vi "DP.vi"(7 "Cluster 2":T1={{[44.26, 44.35, 44.44, 44.4, 44.32, 44.24, 44.13, 44.04, 43.96, 43.84, 43.81, 43.85, 43.72, 43.660000000000004, 43.730000000000004, 43.800000000000004, 43.93, 44.1, 44.22, 44.35, 44.47, 44.59, 44.800000000000004, 44.79, 44.82, 44.9, 45.02, 45.14, 45.35, 45.47, 45.59, 45.72, 45.88, 46.04, 46.0, 46.06, 46.13, 46.26, 46.42, 46.54, 46.67, 46.75, 46.83, 46.96, 47.08, 46.99, 47.03, 47.08, 47.160000000000004, 47.24, 47.32, 47.4, 47.49, 47.57, 47.65, 47.82, 47.730000000000004, 47.76, 47.84, 47.910000000000004, 47.99, 48.06, 48.14, 48.300000000000004, 48.43, 48.550000000000004, 48.67, 48.58, 48.6, 48.660000000000004, 48.75, 48.83, 48.94, 49.03, 49.11, 49.19, 49.27, 49.34, 49.2, 49.19, 49.230000000000004, 49.300000000000004, 49.35, 49.410000000000004, 49.57, 49.620000000000005, 49.660000000000004, 49.74, 49.57, 49.56, 49.58, 49.59, 49.620000000000005, 49.620000000000005, 49.660000000000004, 49.72, 49.75, 49.75, 49.76, 49.63, 49.63, 49.65, 49.65, 49.68, 49.71, 49.75, 49.78, 49.79, 49.870000000000005, 49.86, 49.7, 49.74, 49.75, 49.76, 49.81, 49.81, 49.86, 49.92, 49.97, 49.99, 50.0, 49.86, 49.86], [8.77817e-16, 8.28027e-16, 6.52256e-16, 7.37271e-16, 6.27782e-16, 7.80488e-16, 6.90707e-16, 8.78684e-16, 6.40232e-16, 7.51014e-16, 8.39314e-16, 7.48335e-16, 8.32474e-16, 7.10942e-16, 8.13954e-16, 7.61842e-16, 7.02305e-16, 8.45773e-16, 8.03435e-16, 9.26691e-16, 7.76441e-16, 8.47353e-16, 7.63208e-16, 7.75768e-16, 6.68938e-16, 6.3854e-16, 7.55169e-16, 9.2689e-16, 6.32594e-16, 7.8272e-16, 7.1802e-16, 7.55778e-16, 7.51571e-16, 7.70614e-16, 8.06029e-16, 8.48296e-16, 7.03956e-16, 8.42624e-16, 9.30632e-16, 6.06052e-16, 6.08322e-16, 7.13091e-16, 7.19724e-16, 7.89003e-16, 7.39076e-16, 8.69906e-16, 8.07947e-16, 7.16363e-16, 7.4837e-16, 8.39116e-16, 7.669e-16, 7.29213e-16, 7.26208e-16, 7.54206e-16, 9.32708e-16, 6.57226e-16, 8.41261e-16, 8.58932e-16, 7.73647e-16, 8.51593e-16, 9.21785e-16, 7.29269e-16, 8.09357e-16, 7.50264e-16, 6.81245e-16, 6.31947e-16, 8.77664e-16, 7.8308e-16, 6.85733e-16, 8.74226e-16, 7.71087e-16, 6.79358e-16, 7.5292e-16, 7.27687e-16, 6.37196e-16, 7.75217e-16, 6.21999e-16, 8.42722e-16, 7.84671e-16, 7.54633e-16, 7.64522e-16, 6.04899e-16, 7.18221e-16, 7.30785e-16, 6.70458e-16, 6.68644e-16, 9.06164e-16, 8.8495e-16, 7.79631e-16, 6.61027e-16, 7.21651e-16, 8.56918e-16, 7.49602e-16, 9.56225e-16, 8.38042e-16, 8.06504e-16, 8.60563e-16, 7.40136e-16, 8.40538e-16, 8.35315e-16, 6.48936e-16, 7.08314e-16, 7.77072e-16, 6.66569e-16, 8.04058e-16, 5.94751e-16, 7.63012e-16, 8.0808e-16, 8.87855e-16, 7.52696e-16, 7.48839e-16, 8.42634e-16, 7.77712e-16, 7.77393e-16, 4.45006e-16, 8.08676e-16, 8.80301e-16, 6.99735e-16, 7.18579e-16, 9.3345e-16, 6.93248e-16, 5.1134e-16, 7.0391e-16]}, {[44.26, 44.35, 44.44, 44.4, 44.32, 44.24, 44.13, 44.04, 43.96, 43.84, 43.81, 43.85, 43.72, 43.660000000000004, 43.730000000000004, 43.800000000000004, 43.93, 44.1, 44.22, 44.35, 44.47, 44.59, 44.800000000000004, 44.79, 44.82, 44.9, 45.02, 45.14, 45.35, 45.47, 45.59, 45.72, 45.88, 46.04, 46.0, 46.06, 46.13, 46.26, 46.42, 46.54, 46.67, 46.75, 46.83, 46.96, 47.08, 46.99, 47.03, 47.08, 47.160000000000004, 47.24, 47.32, 47.4, 47.49, 47.57, 47.65, 47.82, 47.730000000000004, 47.76, 47.84, 47.910000000000004, 47.99, 48.06, 48.14, 48.300000000000004, 48.43, 48.550000000000004, 48.67, 48.58, 48.6, 48.660000000000004, 48.75, 48.83, 48.94, 49.03, 49.11, 49.19, 49.27, 49.34, 49.2, 49.19, 49.230000000000004, 49.300000000000004, 49.35, 49.410000000000004, 49.57, 49.620000000000005, 49.660000000000004, 49.74, 49.57, 49.56, 49.58, 49.59, 49.620000000000005, 49.620000000000005, 49.660000000000004, 49.72, 49.75, 49.75, 49.76, 49.63, 49.63, 49.65, 49.65, 49.68, 49.71, 49.75, 49.78, 49.79, 49.870000000000005, 49.86, 49.7, 49.74, 49.75, 49.76, 49.81, 49.81, 49.86, 49.92, 49.97, 49.99, 50.0, 49.86, 49.86], [8.77817e-16, 8.28027e-16, 6.52256e-16, 7.37271e-16, 6.27782e-16, 7.80488e-16, 6.90707e-16, 8.78684e-16, 6.40232e-16, 7.51014e-16, 8.39314e-16, 7.48335e-16, 8.32474e-16, 7.10942e-16, 8.13954e-16, 7.61842e-16, 7.02305e-16, 8.45773e-16, 8.03435e-16, 9.26691e-16, 7.76441e-16, 8.47353e-16, 7.63208e-16, 7.75768e-16, 6.68938e-16, 6.3854e-16, 7.55169e-16, 9.2689e-16, 6.32594e-16, 7.8272e-16, 7.1802e-16, 7.55778e-16, 7.51571e-16, 7.70614e-16, 8.06029e-16, 8.48296e-16, 7.03956e-16, 8.42624e-16, 9.30632e-16, 6.06052e-16, 6.08322e-16, 7.13091e-16, 7.19724e-16, 7.89003e-16, 7.39076e-16, 8.69906e-16, 8.07947e-16, 7.16363e-16, 7.4837e-16, 8.39116e-16, 7.669e-16, 7.29213e-16, 7.26208e-16, 7.54206e-16, 9.32708e-16, 6.57226e-16, 8.41261e-16, 8.58932e-16, 7.73647e-16, 8.51593e-16, 9.21785e-16, 7.29269e-16, 8.09357e-16, 7.50264e-16, 6.81245e-16, 6.31947e-16, 8.77664e-16, 7.8308e-16, 6.85733e-16, 8.74226e-16, 7.71087e-16, 6.79358e-16, 7.5292e-16, 7.27687e-16, 6.37196e-16, 7.75217e-16, 6.21999e-16, 8.42722e-16, 7.84671e-16, 7.54633e-16, 7.64522e-16, 6.04899e-16, 7.18221e-16, 7.30785e-16, 6.70458e-16, 6.68644e-16, 9.06164e-16, 8.8495e-16, 7.79631e-16, 6.61027e-16, 7.21651e-16, 8.56918e-16, 7.49602e-16, 9.56225e-16, 8.38042e-16, 8.06504e-16, 8.60563e-16, 7.40136e-16, 8.40538e-16, 8.35315e-16, 6.48936e-16, 7.08314e-16, 7.77072e-16, 6.66569e-16, 8.04058e-16, 5.94751e-16, 7.63012e-16, 8.0808e-16, 8.87855e-16, 7.52696e-16, 7.48839e-16, 8.42634e-16, 7.77712e-16, 7.77393e-16, 4.45006e-16, 8.08676e-16, 8.80301e-16, 6.99735e-16, 7.18579e-16, 9.3345e-16, 6.93248e-16, 5.1134e-16, 7.0391e-16]}}, 8 "Boolean":bool, 9 "Ring 2":u16(ring), 10 "Ring":u16(ring), 11 "Numeric":u16) -> (0 "XY Graph 2":cluster{dbl[], "Best Gaussian Fit":dbl[]}(graph), 1 "XY Graph":cluster{dbl[], "Array":dbl[]}(graph), 2 "RES_LT":dbl, 3 "RES_CT":dbl, 4 "TCC":dbl)   [LabVIEW 2017]
uses:
  <vilib>/Analysis/NI_AALPro.lvlib
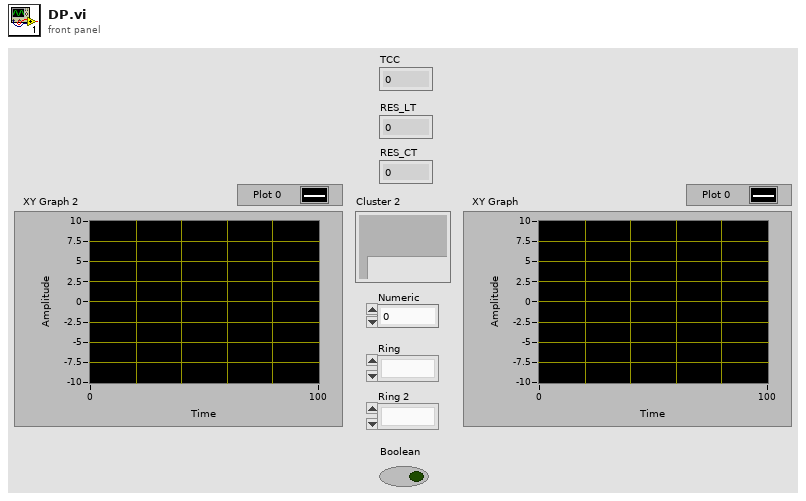
[diagram p1: front panel]
types:
  T1 = cluster{cluster{dbl[], dbl[]}, cluster{dbl[], dbl[]}}
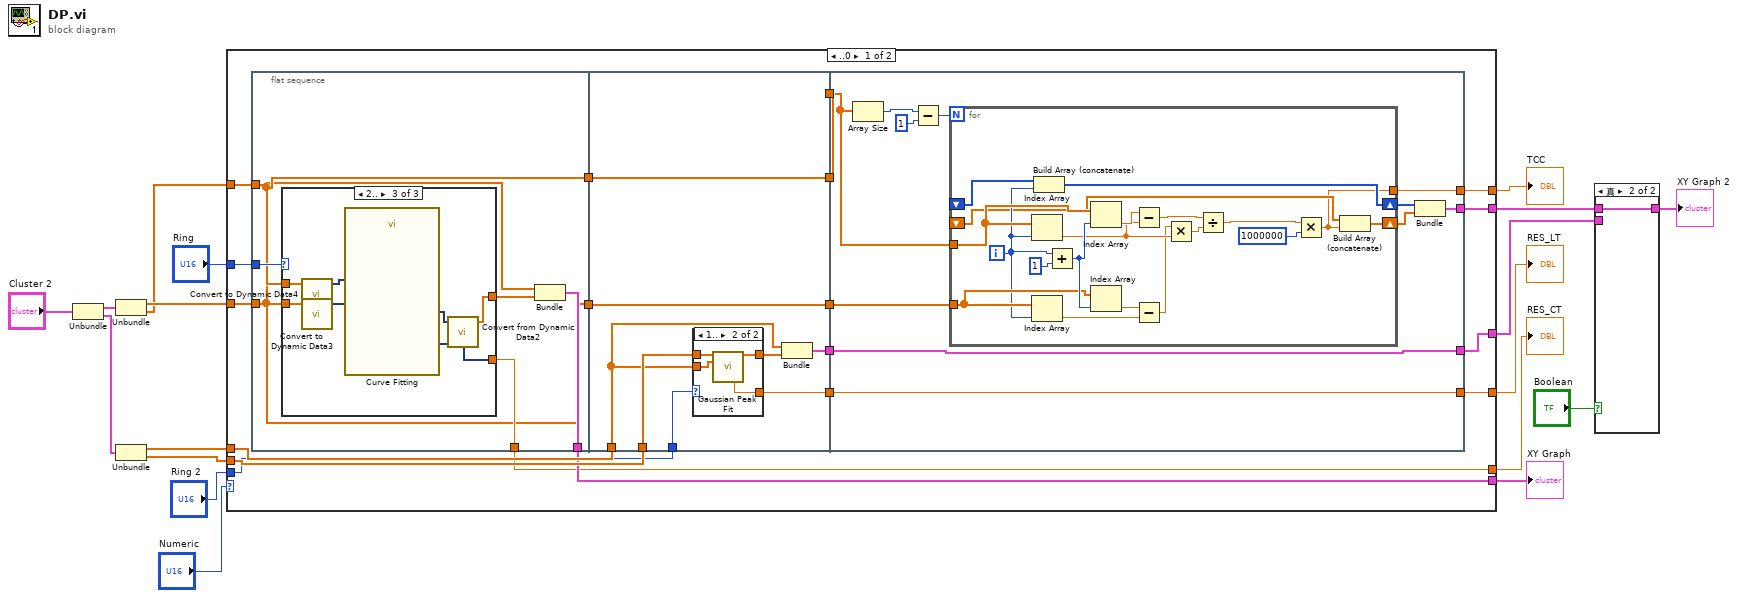
[diagram p0: block diagram]
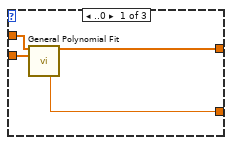
[diagram p3: hidden frame]
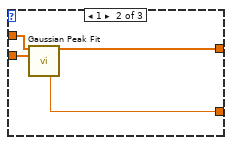
[diagram p4: hidden frame]
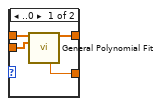
[diagram p5: hidden frame]
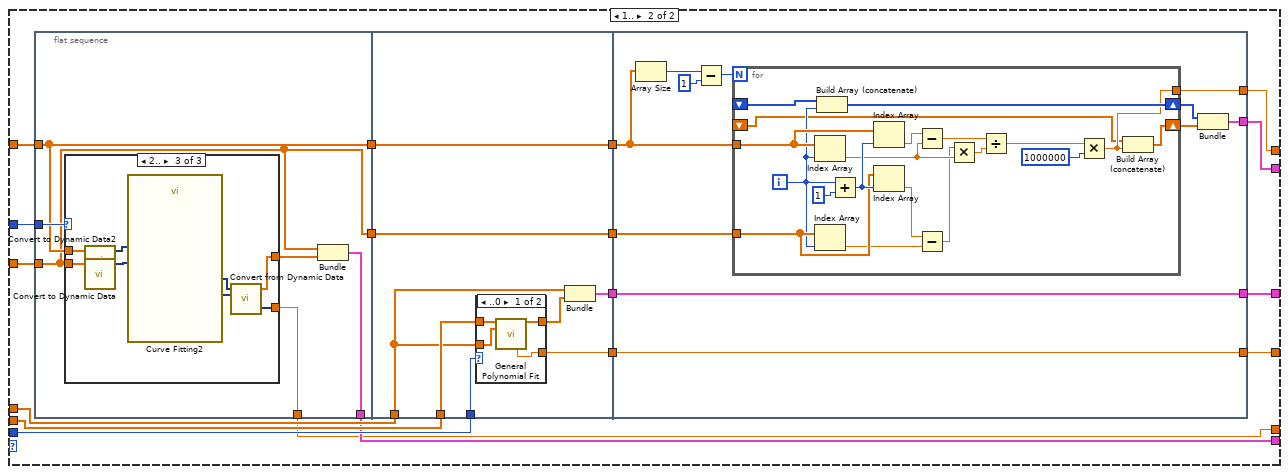
[diagram p6: hidden frame]
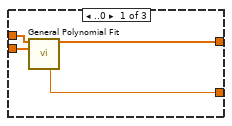
[diagram p7: hidden frame]
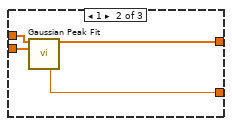
[diagram p8: hidden frame]
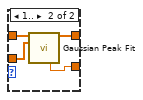
[diagram p9: hidden frame]
diagram:
  n1 = Unbundle("Cluster 2") -> (w16:cluster{dbl[], dbl[]}, w15:cluster{dbl[], dbl[]})
  n2 = Unbundle(w16) -> (w14:dbl[], w13:dbl[])
  n3 = Unbundle(w15) -> (w12:dbl[], w11:dbl[])
  n4 = case shown="..0" "Numeric" {
    tunnel: w14 -> [w35 w121]
    tunnel: w13 -> [w36 w120]
    tunnel: w12 -> [w33 w119]
    tunnel: w11 -> [w34 w118]
    tunnel: "Ring 2" -> [w31 w117]
    tunnel: "Ring" -> [w32 w116]
    tunnel: [w29 w115] -> w3
    tunnel: [w30 w114] -> w8
    tunnel: [w28 w113] -> w7
    tunnel: [w27 w112] -> w6
    tunnel: [w20 w105] -> w5
    tunnel: [w19 w104] -> w2
    frame ..0 {
      n5 = flat-sequence {
        tunnel: w35 -> [w37]
        tunnel: w36 -> [w38]
        tunnel: w32 -> [w42]
        tunnel: [w40] -> w30
        tunnel: [w39] -> w28
        tunnel: [w38] -> w23
        tunnel: [w37] -> w21
        tunnel: w33 -> [w62]
        tunnel: w34 -> [w65]
        tunnel: w31 -> [w64]
        tunnel: [w61] -> w26
        tunnel: [w60] -> w25
        tunnel: [w59] -> w24
        tunnel: w23 -> [w59]
        tunnel: [w58] -> w22
        tunnel: w21 -> [w58]
        tunnel: [w83] -> w27
        tunnel: [w84] -> w29
        tunnel: w26 -> [w84]
        tunnel: w25 -> [w83]
        tunnel: w24 -> [w79]
        tunnel: w22 -> [w78]
        tunnel: [w77] -> w20
        tunnel: [w74] -> w19
        frame #0 {
          n6 = case shown="2.." w42 {
            tunnel: w37 -> [w45 w49 w57]
            tunnel: w38 -> [w46 w50 w55]
            tunnel: [w44 w48 w52] -> w41
            tunnel: [w43 w47 w51] -> w39
            frame ..0 {
              n7 = call <vilib>:"General Polynomial Fit.vi"("Y"=w46, "X"=w45) -> ("Best Polynomial Fit"=w44:dbl[], "residue"=w43:dbl)  [unwired: 10 in, 2 out]
            }
            frame 1 {
              n8 = call <vilib>:"Gaussian Peak Fit.vi"("Y"=w50, "X"=w49) -> ("Best Gaussian Fit"=w48:dbl[], "residue"=w47:dbl)  [unwired: 7 in, 5 out]
            }
            frame 2.. {
              n9 = call "Convert to Dynamic Data4"("Array"=w55) -> ("Dynamic Data Type"=w54:dynamicdata)  [unwired: 3 in]
              n10 = call "Convert to Dynamic Data3"("Array"=w57) -> ("Dynamic Data Type"=w56:dynamicdata)  [unwired: 3 in]
              n11 = call "Curve Fitting"("Locations"=w56, "Signals"=w54) -> ("mean squared error"=w51:dynamicdata, "best fit"=w53:dynamicdata)  [unwired: 5 in, 3 out]
              n12 = call "Convert from Dynamic Data2"("Dynamic Data Type"=w53) -> ("Array"=w52:dbl[])  [unwired: 3 in]
            }
          }
          n13 = Bundle(w37, "Array"=w41) -> (w40:cluster{dbl[], "Array":dbl[]})  [unwired: 1 in]
        }
        frame #1 {
          n14 = case shown="1.." w64 {
            tunnel: w62 -> [w68 w73]
            tunnel: w65 -> [w69 w72]
            tunnel: [w67 w70] -> w63
            tunnel: [w66 w71] -> w60
            frame ..0 {
              n15 = call <vilib>:"General Polynomial Fit.vi"("Y"=w69, "X"=w68) -> ("Best Polynomial Fit"=w67:dbl[], "residue"=w66:dbl)  [unwired: 10 in, 2 out]
            }
            frame 1.. {
              n16 = call <vilib>:"Gaussian Peak Fit.vi"("Y"=w72, "X"=w73) -> ("Best Gaussian Fit"=w70:dbl[], "residue"=w71:dbl)  [unwired: 7 in, 5 out]
            }
          }
          n17 = Bundle(w62, "Best Gaussian Fit"=w63) -> (w61:cluster{dbl[], "Best Gaussian Fit":dbl[]})  [unwired: 1 in]
        }
        frame #2 {
          n18 = Array Size(array=w79) -> (size(s)=w81:i32)
          n19 = Subtract(x=w81, y=1) -> (x-y=w80:i32)
          n20 = for {
            N: w80 -> [_]
            tunnel: w79 -> [w102]
            tunnel: w78 -> [w100]
            tunnel: [w85] -> w77
            shift-right: [w88] -> w75
            shift-left: _ -> [w89]
            shift-right: [w87] -> w76
            shift-left: _ -> [w86]
            i -> [w90]
            n21 = Index Array(array=w102, index=w90) -> (element=w96:dbl)
            n22 = Index Array(array=w100, index=w90) -> (element=w98:dbl)
            n23 = Build Array (concatenate)(w89, w90) -> (w88:i32[])
            n24 = Add(x=w90, y=1) -> (x+y=w101:i32)
            n25 = Index Array(array=w102, index=w101) -> (element=w97:dbl)
            n26 = Index Array(array=w100, index=w101) -> (element=w99:dbl)
            n27 = Subtract(x=w97, y=w96) -> (x-y=w94:dbl)
            n28 = Subtract(x=w99, y=w98) -> (x-y=w95:dbl)
            n29 = Multiply(x=w95, y=w96) -> (x*y=w93:dbl)
            n30 = Divide(x=w94, y=w93) -> (x/y=w92:dbl)
            n31 = Multiply(x=w92, y=1000000) -> (x*y=w85:dbl)
            n32 = Build Array (concatenate)(w86, w85) -> (w87:dbl[])
          }
          n33 = Bundle(w75, w76) -> (w74:cluster{i32[], dbl[]})  [unwired: 1 in]
        }
      }
    }
    frame 1.. {
      n34 = flat-sequence {
        tunnel: w121 -> [w122]
        tunnel: w120 -> [w123]
        tunnel: w116 -> [w127]
        tunnel: [w125] -> w114
        tunnel: [w124] -> w113
        tunnel: [w123] -> w108
        tunnel: [w122] -> w107
        tunnel: w119 -> [w148]
        tunnel: w118 -> [w150]
        tunnel: w117 -> [w149]
        tunnel: [w146] -> w111
        tunnel: [w145] -> w110
        tunnel: [w144] -> w109
        tunnel: w108 -> [w144]
        tunnel: w107 -> [w143]
        tunnel: [w143] -> w106
        tunnel: [w168] -> w112
        tunnel: [w169] -> w115
        tunnel: w111 -> [w169]
        tunnel: w110 -> [w168]
        tunnel: w109 -> [w167]
        tunnel: w106 -> [w163]
        tunnel: [w162] -> w105
        tunnel: [w159] -> w104
        frame #0 {
          n35 = case shown="2.." w127 {
            tunnel: w122 -> [w130 w134 w142]
            tunnel: w123 -> [w131 w135 w140]
            tunnel: [w129 w133 w137] -> w126
            tunnel: [w128 w132 w136] -> w124
            frame ..0 {
              n36 = call <vilib>:"General Polynomial Fit.vi"("Y"=w131, "X"=w130) -> ("Best Polynomial Fit"=w129:dbl[], "residue"=w128:dbl)  [unwired: 10 in, 2 out]
            }
            frame 1 {
              n37 = call <vilib>:"Gaussian Peak Fit.vi"("Y"=w135, "X"=w134) -> ("Best Gaussian Fit"=w133:dbl[], "residue"=w132:dbl)  [unwired: 7 in, 5 out]
            }
            frame 2.. {
              n38 = call "Convert to Dynamic Data2"("Array"=w140) -> ("Dynamic Data Type"=w139:dynamicdata)  [unwired: 3 in]
              n39 = call "Convert to Dynamic Data"("Array"=w142) -> ("Dynamic Data Type"=w141:dynamicdata)  [unwired: 3 in]
              n40 = call "Curve Fitting2"("Locations"=w141, "Signals"=w139) -> ("residual"=w136:dynamicdata, "best fit"=w138:dynamicdata)  [unwired: 5 in, 3 out]
              n41 = call "Convert from Dynamic Data"("Dynamic Data Type"=w138) -> ("Array"=w137:dbl[])  [unwired: 3 in]
            }
          }
          n42 = Bundle(w122, "Array"=w126) -> (w125:cluster{dbl[], "Array":dbl[]})  [unwired: 1 in]
        }
        frame #1 {
          n43 = case shown="..0" w149 {
            tunnel: w148 -> [w153 w158]
            tunnel: w150 -> [w154 w157]
            tunnel: [w152 w156] -> w147
            tunnel: [w151 w155] -> w145
            frame ..0 {
              n44 = call <vilib>:"General Polynomial Fit.vi"("Y"=w154, "X"=w153) -> ("Best Polynomial Fit"=w152:dbl[], "residue"=w151:dbl)  [unwired: 10 in, 2 out]
            }
            frame 1.. {
              n45 = call <vilib>:"Gaussian Peak Fit.vi"("Y"=w157, "X"=w158) -> ("Best Gaussian Fit"=w156:dbl[], "residue"=w155:dbl)  [unwired: 7 in, 5 out]
            }
          }
          n46 = Bundle(w148, "Best Gaussian Fit"=w147) -> (w146:cluster{dbl[], "Best Gaussian Fit":dbl[]})  [unwired: 1 in]
        }
        frame #2 {
          n47 = Array Size(array=w167) -> (size(s)=w165:i32)
          n48 = Subtract(x=w165, y=1) -> (x-y=w164:i32)
          n49 = for {
            N: w164 -> [_]
            tunnel: w167 -> [w187]
            tunnel: w163 -> [w185]
            tunnel: [w172] -> w162
            shift-right: [w175] -> w160
            shift-left: _ -> [w174]
            shift-right: [w171] -> w161
            shift-left: _ -> [w170]
            i -> [w173]
            n50 = Index Array(array=w187, index=w173) -> (element=w181:dbl)
            n51 = Index Array(array=w185, index=w173) -> (element=w183:dbl)
            n52 = Build Array (concatenate)(w174, w173) -> (w175:i32[])
            n53 = Add(x=w173, y=1) -> (x+y=w186:i32)
            n54 = Index Array(array=w187, index=w186) -> (element=w182:dbl)
            n55 = Index Array(array=w185, index=w186) -> (element=w184:dbl)
            n56 = Subtract(x=w182, y=w181) -> (x-y=w179:dbl)
            n57 = Subtract(x=w184, y=w183) -> (x-y=w180:dbl)
            n58 = Multiply(x=w180, y=w181) -> (x*y=w178:dbl)
            n59 = Divide(x=w179, y=w178) -> (x/y=w177:dbl)
            n60 = Multiply(x=w177, y=1000000) -> (x*y=w172:dbl)
            n61 = Build Array (concatenate)(w170, w172) -> (w171:dbl[])
          }
          n62 = Bundle(w160, w161) -> (w159:cluster{i32[], dbl[]})  [unwired: 1 in]
        }
      }
    }
  }
  "XY Graph" <- w8
  "RES_CT" <- w7
  "RES_LT" <- w6
  "TCC" <- w5
  n63 = case shown="真" "Boolean" {
    tunnel: [w189 w190] -> w4
    tunnel: w3 -> [w189 _]
    tunnel: w2 -> [_ w190]
    frame False {
    }
    frame True {
    }
  }
  "XY Graph 2" <- w4
